vi "Update Calibration Constants.vi"(8 "error in":errorcluster, 11 "cPAS in":refnum<class "cPAS.lvclass">) -> (0 "error out":errorcluster, 3 "cPAS out":refnum<class "cPAS.lvclass">)   [LabVIEW 2015, in "cPAS.lvclass"]
doc: "Check for an update on the conversion constants for IA to absorption."
uses:
  cPAS.lvclass
  Reusable/PAS/Main/Read Cells.vi
  Reusable/PAS/Cell/Write extParams.vi
  Reusable/PAS/Main/Write Cells.vi
  Reusable/PAS/Cell/PAS Cell.lvclass
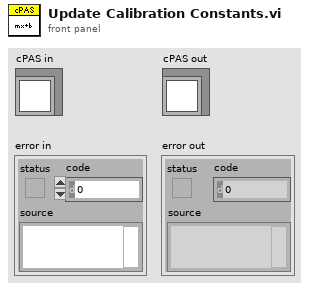
[diagram p1: front panel]
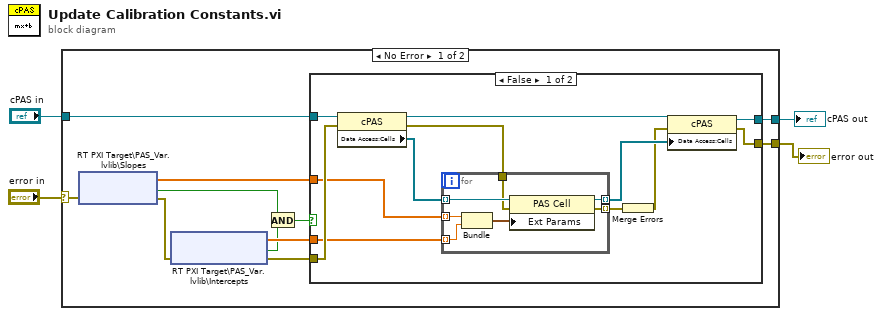
[diagram p0: block diagram]
diagram:
  n1 = case shown="No Error" "error in" {
    selector: "error in" -> [w7 w38]
    tunnel: [w13 w38] -> w3
    tunnel: [w14 w37] -> w1
    tunnel: "cPAS in" -> [w15 w37]
    frame No Error {
      n2 = shared-variable "RT PXI Target\\PAS_Var.lvlib\\Slopes"(error in=w7) -> (w11:sgl[], error out=w6:errorcluster, w9:bool)  [unwired: 1 in]
      n3 = shared-variable "RT PXI Target\\PAS_Var.lvlib\\Intercepts"(error in=w6) -> (w10:sgl[], error out=w5:errorcluster, w8:bool)  [unwired: 1 in]
      n4 = And(x=w9, y=w8) -> (x .and. y?=w12:bool)
      n5 = case shown="False" w12 {
        tunnel: w15 -> [w27 w36]
        tunnel: [w25 w36] -> w14
        tunnel: w5 -> [w20 w35]
        tunnel: [w18 w35] -> w13
        tunnel: w11 -> [w17 _]
        tunnel: w10 -> [w16 _]
        frame False {
          n6 = property class="cPAS"(reference=w27, error in=w20) -> (reference out=w24:refnum<class "cPAS.lvclass">, error out=w19:errorcluster, "Data Access:Cells"=w26:refnum<class "PAS Cell.lvclass">[])
          n7 = for {
            tunnel: w26 -> [w34] mode=indexing
            tunnel: [w33] -> w23 mode=indexing
            tunnel: [w32] -> w22 mode=indexing
            tunnel: w19 -> [w31]
            tunnel: w17 -> [w29] mode=indexing
            tunnel: w16 -> [w28] mode=indexing
            n8 = Bundle("Numeric"=w29, "Numeric"=w28) -> (w30:cluster{"Numeric":sgl, "Numeric":sgl})  [unwired: 1 in]
            n9 = property class="PAS Cell"(reference=w34, error in=w31, "Ext Params"=w30) -> (reference out=w33:refnum<class "PAS Cell.lvclass">, error out=w32:errorcluster)
          }
          n10 = Merge Errors(w22) -> (w21:errorcluster)
          n11 = property class="cPAS"(reference=w24, error in=w21, "Data Access:Cells"=w23) -> (reference out=w25:refnum<class "cPAS.lvclass">, error out=w18:errorcluster)
        }
        frame True {
        }
      }
    }
    frame Error {
    }
  }
  "error out" <- w3
  "cPAS out" <- w1
